vi "Data.Write.vi"(7 "ingore UI update (F)":bool, 8 "error in":errorcluster, 9 "priority":bool, 10 "data value":T1, 11 "DVR.state":T2) -> (0 "error out":errorcluster)   [LabVIEW 2020]
uses:
  _controls/state.ctl
  7526ba03-708b-410e-8304-4a6dc7be2616.vi
  _controls/data.ref.ctl
  _controls/data.ctl
  _controls/data.vars.ctl
  _controls/flip.ctl
  <vilib>/vision/Image Controls.llb/IMAQ Image.ctl
  camera/camera.lvclass
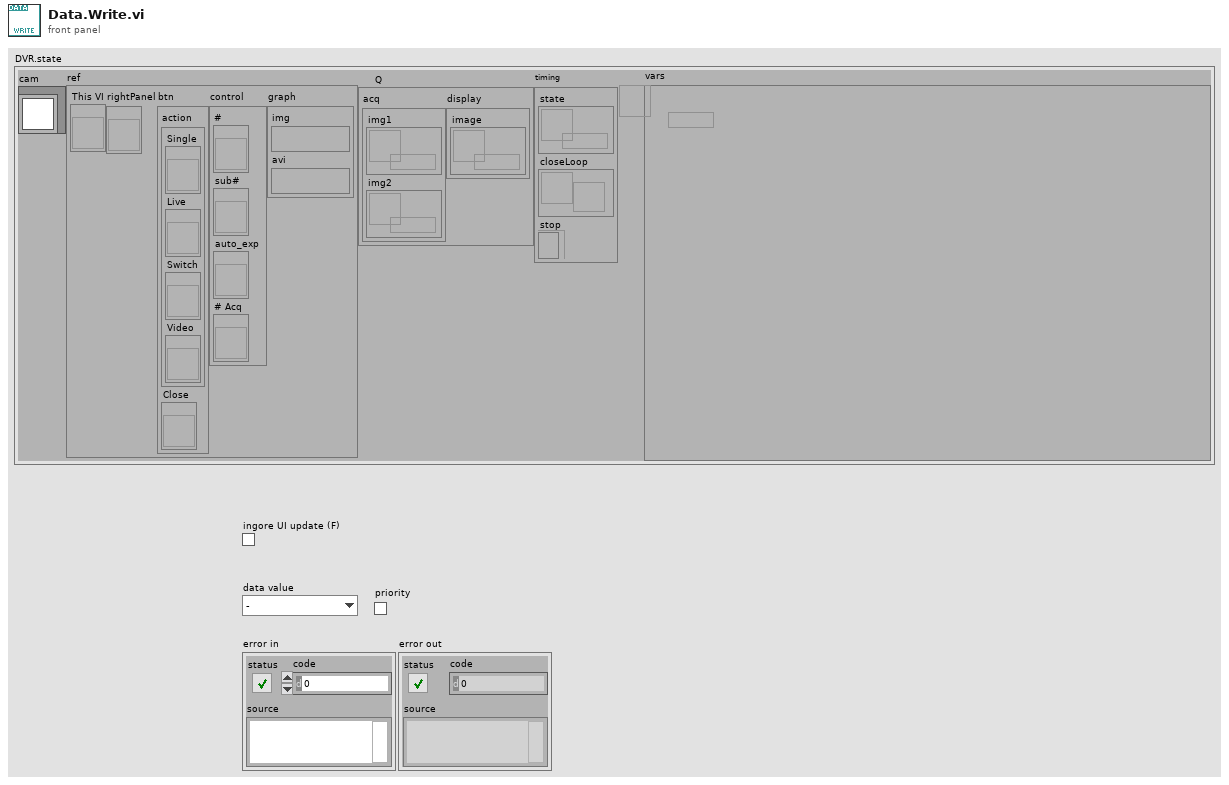
[diagram p1: front panel]
types:
  T1 = typedef "state.ctl" = enum16{"-", "single", "video", "livePL", "PL"}
  T2 = typedef "data.ctl" = cluster{"cam":refnum<class "camera.lvclass">, "ref":T3, "Q":cluster{"acq":cluster{"img1":refnum<queue>, "img2":refnum<queue>}, "display":cluster{"image":refnum<queue>}}, "timing":cluster{"state":refnum<queue>, "closeLoop":refnum<notifier>, "stop":refnum<k4>}, "vars":refnum<data-value>}
  T3 = typedef "data.ref.ctl" = cluster{"This VI":refnum<vi>, "rightPanel":refnum<vi>, "btn":cluster{"action":cluster{"Single":refnum<vi>, "Live":refnum<vi>, "Switch":refnum<vi>, "Video":refnum<vi>}, "Close":refnum<vi>}, "control":cluster{"#":refnum<vi>, "sub#":refnum<vi>, "auto_exp":refnum<vi>, "# Acq":refnum<vi>}, "graph":cluster{"img":T4, "avi":T4}}
  T4 = typedef "IMAQ Image.ctl" = refnum<image>
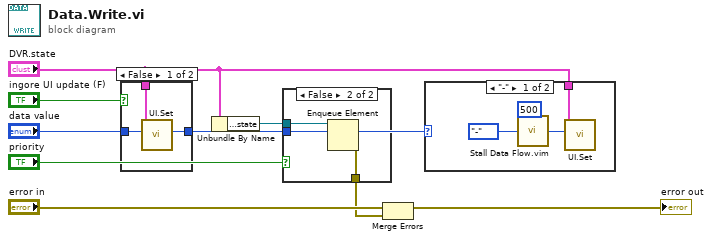
[diagram p0: block diagram]
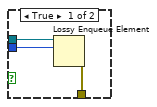
[diagram p3: hidden frame]
diagram:
  n1 = case shown="False" "ingore UI update (F)" {
    tunnel: "data value" -> [w10 w12]
    tunnel: "DVR.state" -> [w11 _]
    tunnel: [w10 w12] -> w2
    frame False {
      n2 = call "UI.Set.vi"("data value"=w10, "DVR.state"=w11) -> ()  [unwired: 10 in]
    }
    frame True {
    }
  }
  n3 = Unbundle By Name("DVR.state") -> ("timing.state"=w6:refnum<queue>)
  n4 = case shown="False" "priority" {
    tunnel: [w15 w18] -> w7
    tunnel: w6 -> [w13 w16]
    tunnel: w2 -> [w14 w17]
    frame True {
      n5 = Lossy Enqueue Element(queue=w13, element=w14) -> (error out=w15:errorcluster)  [unwired: 1 in, 3 out]
    }
    frame False {
      n6 = Enqueue Element(queue=w16, element=w17) -> (error out=w18:errorcluster)  [unwired: 2 in, 2 out]
    }
  }
  n7 = Merge Errors("error in", w7) -> (→"error out":errorcluster)
  n8 = case shown="\"stop\"" w2 {
    tunnel: "DVR.state" -> [w22 _]
    frame "-" {
      n9 = call "Stall Data Flow.vim"("value in"=state."-" ("data value"), "milliseconds to wait"=u32 500) -> ("value out"=w20:T1)  [unwired: 1 out]
      n10 = call "UI.Set.vi"("data value"=w20, "DVR.state"=w22) -> ()  [unwired: 10 in]
    }
    frame Default {
    }
  }
